vi "SeqMgr.1D Array, Read Item.vi"(8 "error in":errorcluster, 10 "ArrayVarName":string, 11 "Data1D":variant) -> (0 "error out":errorcluster, 2 "Value":string, 3 "Data1D Dup":variant)   [LabVIEW 2024, in "EQMF.lvlib" / "SeqMgr.lvlib"]
uses:
  SeqMgr.lvlib
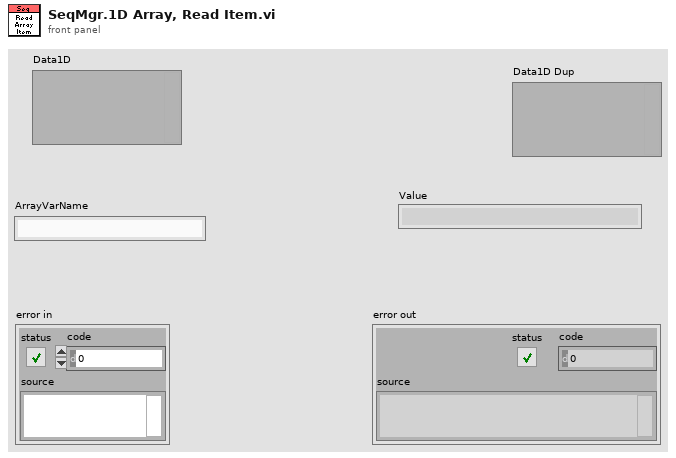
[diagram p1: front panel]
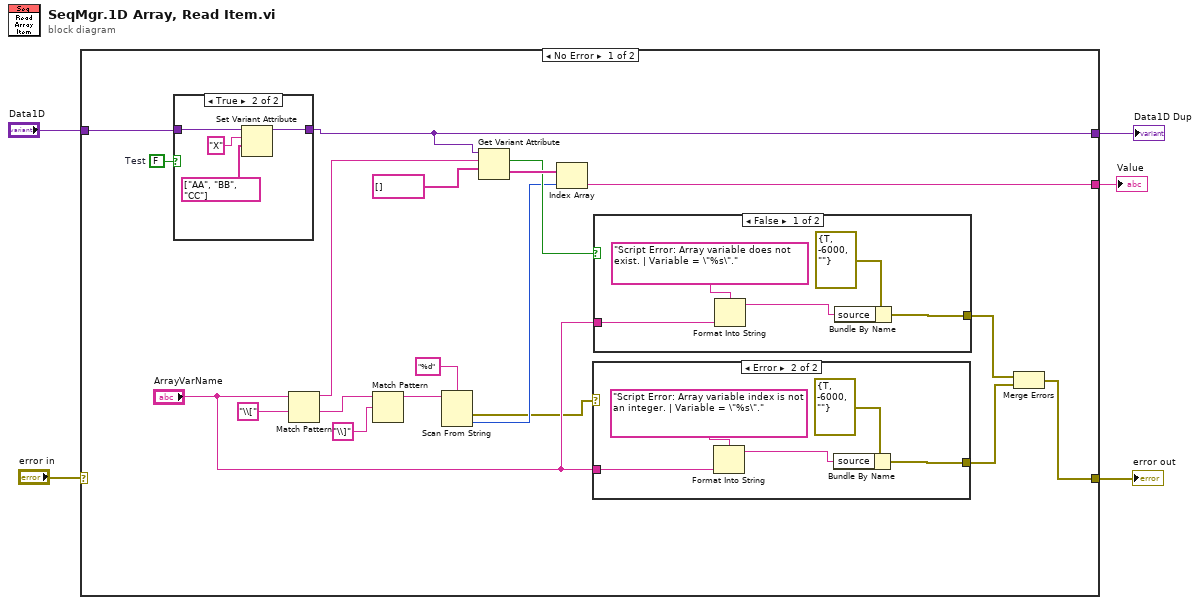
[diagram p0: block diagram]
diagram:
  n1 = case shown="No Error" "error in" {
    selector: "error in" -> [_ w41]
    tunnel: [w22 _] -> w5
    tunnel: [w10 w41] -> w3
    tunnel: [w7 w40] -> w2
    tunnel: "Data1D" -> [w6 w40]
    frame No Error {
      w9 = FALSE  # Test
      n2 = case shown="True" w9 {
        tunnel: w6 -> [w25 w29]
        tunnel: [w25 w28] -> w7
        frame False {
        }
        frame True {
          n3 = Set Variant Attribute(Variant=w29, name="X" ("String"), value=string[] ["AA", "BB", "CC"] ("Data")) -> (Variant out=w28:variant)  [unwired: 1 in, 2 out]
        }
      }
      n4 = Match Pattern(string="ArrayVarName", regular expression="\\[") -> (before substring=w14:string, after substring=w20:string)  [unwired: 1 in, 2 out]
      n5 = Match Pattern(string=w20, regular expression="\\]") -> (before substring=w17:string)  [unwired: 1 in, 3 out]
      n6 = Scan From String(format string="%d", input string=w17) -> (error out=w8:errorcluster, output 1=w15:i32)  [unwired: 3 in, 2 out]
      n7 = Get Variant Attribute(Variant=w7, name=w14, default value (empty Variant)=string[] [] ("Data")) -> (found=w16:bool, value=w23:string[])  [unwired: 1 in, 2 out]
      n8 = Index Array(array=w23, index=w15) -> (element=w22:string)
      n9 = case shown="Error" w8 {
        tunnel: "ArrayVarName" -> [_ w33]
        tunnel: [_ w30] -> w11
        frame No Error {
        }
        frame Error {
          n10 = Format Into String(format string="Script Error: Array variable index is not an integer. | Variable = \"%s\".", w33) -> (resulting string=w31:string)  [unwired: 2 in, 1 out]
          n11 = Bundle By Name(cluster=errorcluster {"status"=TRUE, "code"=-6000, "source"=""} ("error constant"), "source"=w31) -> (w30:errorcluster)
        }
      }
      n12 = case shown="False" w16 {
        tunnel: "ArrayVarName" -> [w38 _]
        tunnel: [w35 _] -> w13
        frame False {
          n13 = Format Into String(format string="Script Error: Array variable does not exist. | Variable = \"%s\".", w38) -> (resulting string=w36:string)  [unwired: 2 in, 1 out]
          n14 = Bundle By Name(cluster=errorcluster {"status"=TRUE, "code"=-6000, "source"=""} ("error constant"), "source"=w36) -> (w35:errorcluster)
        }
        frame True {
        }
      }
      n15 = Merge Errors(w13, w11) -> (w10:errorcluster)
    }
    frame Error {
    }
  }
  "Value" <- w5
  "error out" <- w3
  "Data1D Dup" <- w2
